vi "Write Timeout.vi"(8 "Error In":errorcluster) -> (0 "Error Out":errorcluster)   [LabVIEW 2018, in "Tests.lvlib" / "Session.lvlib"]
uses:
  Session.lvlib
  src/Toolkit/Session/Support/Create from SSH.vi
  src/Toolkit/Session/Support/Destroy to SSH.vi
  <vilib>/addons/_JKI Toolkits/Caraya/classes/Test/Test.lvclass
  src/Toolkit/SSH/SSH.lvclass
  src/Toolkit/Session/Session.lvclass
  <vilib>/addons/_JKI Toolkits/Caraya/classes/Assert/Assert.lvclass
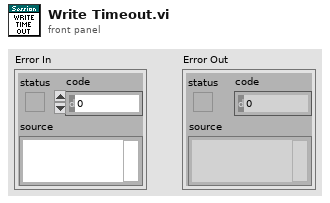
[diagram p1: front panel]
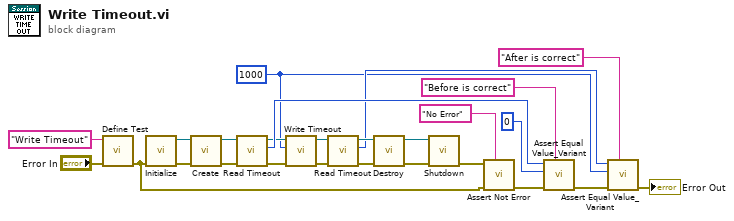
[diagram p0: block diagram]
diagram:
  w2 = 1000 ("Timeout")
  n1 = call <vilib>:"Define Test.vi"("error in (no error)"="Error In", "Label (VI Title)"="Write Timeout") -> ("error out"=w18:errorcluster)  [unwired: 9 in]
  n2 = call "Initialize.vi"("Error In"=w18) -> ("Error Out"=w24:errorcluster, "SSH"=w23:refnum<class "SSH.lvclass">)  [unwired: 9 in]
  n3 = call-poly "Create.vi"("Error In"=w24, "SSH"=w23) -> ("Error Out"=w14:errorcluster, "Sesssion"=w15:refnum<class "Session.lvclass">)  [unwired: 8 in]
  n4 = call "Read Timeout.vi"("Error In"=w14, "Session In"=w15) -> ("Error Out"=w10:errorcluster, "Timeout"=w13:i32, "Sesssion Out"=w11:refnum<class "Session.lvclass">)  [unwired: 7 in]
  n5 = call "Write Timeout.vi"("Error In"=w10, "Timeout"=w2, "Session In"=w11) -> ("Error Out"=w8:errorcluster, "Sesssion Out"=w9:refnum<class "Session.lvclass">)  [unwired: 7 in]
  n6 = call "Read Timeout.vi"("Error In"=w8, "Session In"=w9) -> ("Error Out"=w7:errorcluster, "Timeout"=w3:i32, "Sesssion Out"=w6:refnum<class "Session.lvclass">)  [unwired: 7 in]
  n7 = call-poly "Destroy.vi"("Error In"=w7, "Session"=w6) -> ("Error Out"=w21:errorcluster, "SSH"=w22:refnum<class "SSH.lvclass">)  [unwired: 8 in]
  n8 = call "Shutdown.vi"("Error In"=w21, "SSH"=w22) -> ("Error Out"=w20:errorcluster)  [unwired: 9 in]
  n9 = call <vilib>:"Assert Not Error.vi"("Label"="No Error", "error in (no error)"=w18, "Not Error?"=w20) -> ("error out"=w17:errorcluster)  [unwired: 8 in]
  n10 = call <vilib>:"Assert Equal Value_Variant.vi"("Label"="Before is correct", "error in (no error)"=w17, "Y"=0 ("Timeout"), "X"=w13) -> ("error out"=w5:errorcluster)  [unwired: 7 in]
  n11 = call <vilib>:"Assert Equal Value_Variant.vi"("Label"="After is correct", "error in (no error)"=w5, "Y"=w2, "X"=w3) -> ("error out"=→"Error Out":errorcluster)  [unwired: 7 in]
